vi "Get File LV Version.vi"(0 "Path":path) -> (2 "LV Version":u32)   [LabVIEW 2019, in "Caraya Library.lvlib" / "Caraya Item.lvclass"]
uses:
  Caraya Item.lvclass
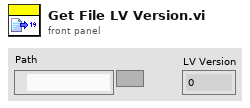
[diagram p1: front panel]
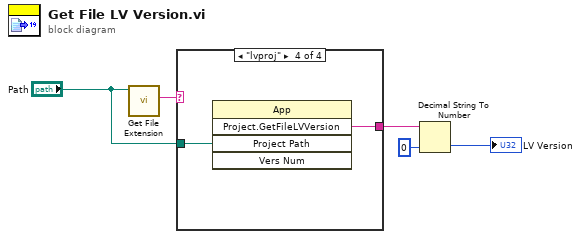
[diagram p0: block diagram]
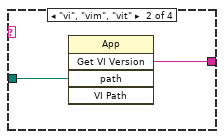
[diagram p3: hidden frame]
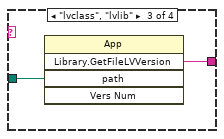
[diagram p4: hidden frame]
diagram:
  n1 = call <vilib>:"Get File Extension.vi"("file"="Path") -> ("lowercase file extension"=w3:string)  [unwired: 6 in, 4 out]
  n2 = case shown="\"lvproj\"" w3 {
    tunnel: "Path" -> [_ w7 w8 w11]
    tunnel: [_ w6 w9 w10] -> w2
    frame Default {
    }
    frame "vi", "vim", "vit" {
      n3 = invoke class="App" method="Get VI Version"("path"=w7) -> ("GetVIVers"=w6:string)  [unwired: 4 in, 4 out]
    }
    frame "lvclass", "lvlib" {
      n4 = invoke class="App" method="Library.GetFileLVVersion"("path"=w8) -> ("Library.GetFileLVVersion"=w9:string)  [unwired: 4 in, 4 out]
    }
    frame "lvproj" {
      n5 = invoke class="App" method="Project.GetFileLVVersion"("Project Path"=w11) -> ("Project.GetFileLVVersion"=w10:string)  [unwired: 4 in, 4 out]
    }
  }
  n6 = Decimal String To Number(string=w2, default (0L)=u32 0 ("default (0 I32)")) -> (number=→"LV Version":u32)  [unwired: 1 in, 1 out]
